vi "Inverse Matrix.vi"   [LabVIEW 2014, in "NI_AALBase.lvlib"]
doc: "Finds <B>Inverse Matrix</B>, if it exists, of <B>Input Matrix</B>. Wire data to the <B>Input Matrix</B> input to determine the polymorphic instance to use or manually select the instance."
uses:
  NI_AALBase.lvlib
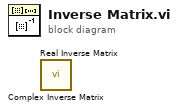
[diagram p0: block diagram]
diagram:
  n1 = call "Complex Inverse Matrix.vi"() -> ()  [unwired: 2 in, 2 out]
  n2 = call "Real Inverse Matrix.vi"() -> ()  [unwired: 2 in, 2 out]
